vi "Configure Items To Log.vi"(8 "error in (no error)":errorcluster, 10 "Items To Log":bool[](array[boolean])=[TRUE, TRUE, TRUE, TRUE, TRUE, TRUE, TRUE, TRUE, TRUE, TRUE, TRUE, TRUE, TRUE, TRUE, TRUE, TRUE, TRUE, TRUE], 11 "VISA resource name":refnum<visa-resource-name>) -> (0 "error out":errorcluster, 3 "VISA resource name out":refnum<visa-resource-name>)   [LabVIEW 2013, in "Watts Up Series.lvlib"]
doc: "Configures the values that the Watts Up meter will log. Values not enabled will not be logged internally or remotely (if using the .NET device).\n\n<b>WARNING 1:</b> Changing which items are logged will clear the meter's internal memory. You may wish to save your data before proceeding. \n\n<b>WARNING 2:</b> Setting all items to log to OFF will cause the Watts Up device to freeze and communication with it cannot be restored until the meter's power is recycled."
uses:
  <instrlib>/Watts Up Series/Watts Up Series.lvlib
panel:
  # "Watts"
  # "Volts"
  # "Amps"
  # "Watt Hours"
  # "Cost"
  # "WH/Month"
  # "Cost/Month"
  # "Wmax"
  # "Vmax"
  # "Amax"
  # "Wmin"
  # "Vmin"
  # "Amin"
  # "Power Factor"
  # "Duty Cycle"
  # "Power Cycle"
  # "Line Freq."
  # "Volt-Amps"
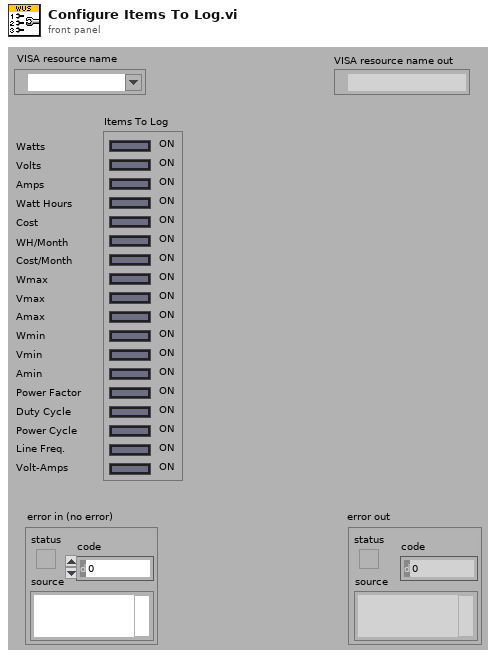
[diagram p1: front panel]
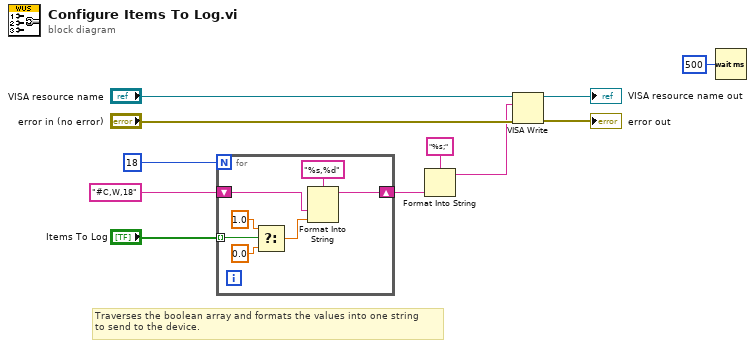
[diagram p0: block diagram]
diagram:
  # "Traverses the boolean array and formats the values into one string\nto send to the device."
  n1 = for {
    N: 18 -> [_]
    tunnel: "Items To Log" -> [w18] mode=indexing
    shift-right: [w12] -> w4
    shift-left: "#C,W,18" -> [w14]
    n2 = Select(t=1.0, s=w18, f=0.0) -> (s? t:f=w15:dbl)
    n3 = Format Into String(format string="%s,%d", w14, w15) -> (resulting string=w12:string)  [unwired: 2 in, 1 out]
  }
  n4 = Format Into String(format string="%s;", w4) -> (resulting string=w2:string)  [unwired: 2 in, 1 out]
  n5 = VISA Write(VISA resource name="VISA resource name", write buffer=w2, error in (no error)="error in (no error)") -> (VISA resource name out=→"VISA resource name out":refnum<visa-resource-name>, error out=→"error out":errorcluster)  [unwired: 1 out]
  n6 = Wait (ms)(milliseconds to wait=u32 500) -> ()  [unwired: 1 out]
